vi "Is DQMH Request QD.vi"(8 "error in (no error)":errorcluster, 11 "VI in":refnum<vi>) -> (0 "error out":errorcluster, 2 "Is a DQMH Request":bool, 3 "VI out":refnum<vi>)   [LabVIEW 2017]
doc: "Checks if the SubVI is a DQMH Request or a Request and Wait for Reply."
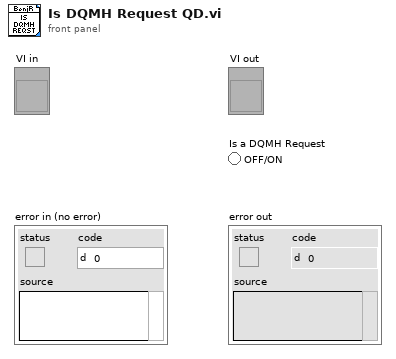
[diagram p1: front panel]
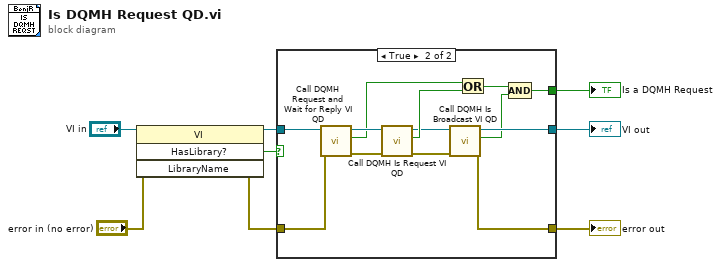
[diagram p0: block diagram]
diagram:
  n1 = invoke class="VI" method="HasLibrary?"(reference="VI in", error in="error in (no error)") -> (reference out=w5:refnum<vi>, error out=w3:errorcluster, "Has Library?"=w4:bool)  [unwired: 2 in, 1 out]
  n2 = case shown="True" w4 {
    tunnel: w5 -> [w9 w22]
    tunnel: w3 -> [w10 w20]
    tunnel: [w10 w14] -> w8
    tunnel: [w9 w16] -> w6
    tunnel: [_ w11] -> w2
    frame False {
    }
    frame True {
      n3 = call "Call DQMH Request and Wait for Reply VI QD.vi"("error in (no error)"=w20, "Request VI in"=w22) -> ("error out"=w21:errorcluster, "Is Request and Wait for Reply"=w18:bool, "Request VI out"=w23:refnum<vi>)  [unwired: 7 in]
      n4 = call "Call DQMH Is Request VI QD.vi"("error in (no error)"=w21, "Request VI in"=w23) -> ("error out"=w15:errorcluster, "Is Request"=w19:bool, "Request VI out"=w17:refnum<vi>)  [unwired: 7 in]
      n5 = call "Call DQMH Is Broadcast VI QD.vi"("error in (no error)"=w15, "Request VI in"=w17) -> ("error out"=w14:errorcluster, "Is Broadcast"=w12:bool, "Request VI out"=w16:refnum<vi>)  [unwired: 7 in]
      n6 = Or(x=w18, y=w19) -> (x .or. y?=w13:bool)
      n7 = Compound Arithmetic op=AND(w13, w12) -> (w11:bool)
    }
  }
  "Is a DQMH Request" <- w2
  "error out" <- w8
  "VI out" <- w6
